vi "Reset Edit Memory.vi"(8 "error in (no error)":errorcluster, 9 "trace name":string, 10 "points":dbl, 11 "VISA resource name":refnum<visa-resource-name>) -> (0 "error out":errorcluster, 3 "VISA resource name out":refnum<visa-resource-name>)   [LabVIEW 2009, in "Tektronix AFG 3000 Series.lvlib"]
doc: "Resets the contents of the edit memory of a Tektronix AFG 3000 series function generator. If a number of points is passed (2-131072), the edit memory is set to that length with each value initialized to the default (8191).\n\nIf a number of points is not provided but a trace name is, then the specified waveform data is copied to edit memory.\n\nIf neither are provided, the edit memory is initialized to the default length (1000) and value (8191)."
uses:
  Tektronix AFG 3000 Series.lvlib
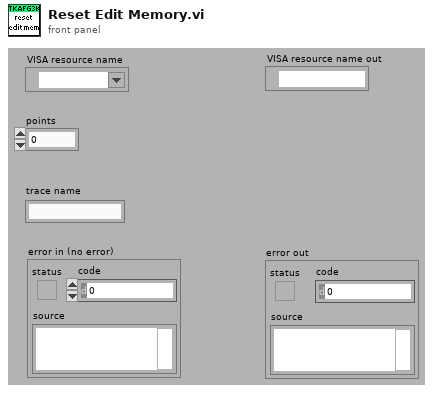
[diagram p1: front panel]
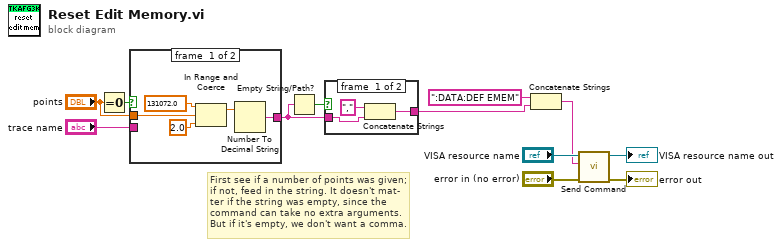
[diagram p0: block diagram]
diagram:
  # "First see if a number of points was given;\nif not, feed in the string. It doesn't mat-\nter if the string was empty, since the\ncommand can take no extra arguments.\nBut if it's empty, we don't want a comma."
  n1 = Equal To 0?(x="points") -> (x = 0?=w9:bool)
  n2 = case shown="False" w9 {
    tunnel: "trace name" -> [_ w18]
    tunnel: "points" -> [w17 _]
    tunnel: [w13 w18] -> w3
    frame #0 {
      n3 = In Range and Coerce(upper limit=131072.0, x=w17, lower limit=2.0) -> (coerced(x)=w14:dbl)  [unwired: 1 out]
      n4 = Number To Decimal String(number=w14) -> (decimal integer string=w13:string)  [unwired: 1 out]
    }
    frame #1 {
    }
  }
  n5 = Empty String/Path?(string/path=w3) -> (empty?=w4:bool)
  n6 = case shown="False" w4 {
    tunnel: w3 -> [w20 w22]
    tunnel: [w19 w22] -> w2
    frame #0 {
      n7 = Concatenate Strings("," ("string"), w20) -> (w19:string)
    }
    frame #1 {
    }
  }
  n8 = Concatenate Strings(":DATA:DEF EMEM" ("string"), w2) -> (w1:string)
  n9 = call "Send Command.vi"("error in (no error)"="error in (no error)", "write buffer"=w1, "VISA resource name"="VISA resource name") -> ("error out"=→"error out":errorcluster, "VISA resource name out"=→"VISA resource name out":refnum<visa-resource-name>)  [unwired: 7 out]
